vi "torque-write (SubVI).vi"(10 "Torque":i16, 11 "ID":u8) -> (3 "result string":string)   [LabVIEW 2017]
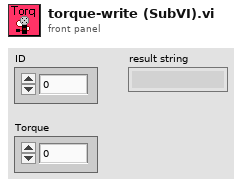
[diagram p1: front panel]
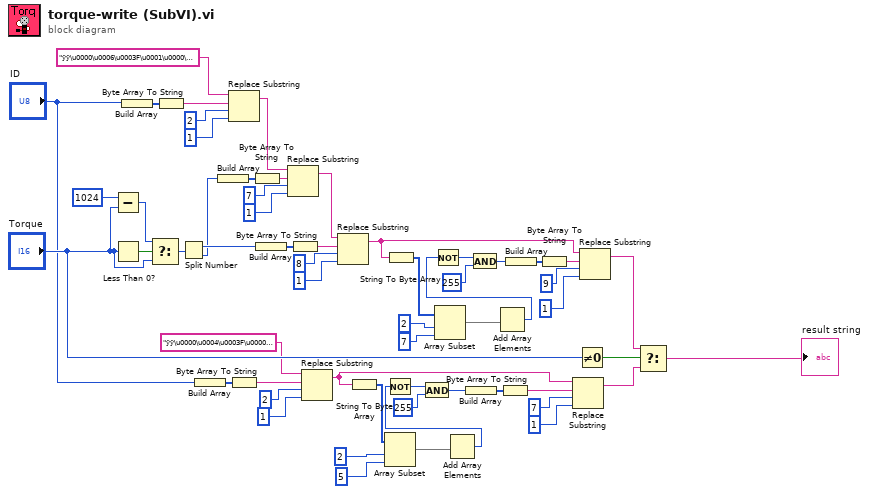
[diagram p0: block diagram]
diagram:
  n1 = Subtract(x=i16 1024, y="Torque") -> (x-y=w34:i16)
  n2 = Less Than 0?(x="Torque") -> (x < 0?=w29:bool)
  n3 = Build Array("ID") -> (w9:u8[])
  n4 = Select(t=w34, s=w29, f="Torque") -> (s? t:f=w31:i16)
  n5 = Byte Array To String(unsigned byte array=w9) -> (string=w8:string)
  n6 = Split Number(x=w31) -> (hi(x)=w33:u8, lo(x)=w32:u8)
  n7 = Build Array("ID") -> (w49:u8[])
  n8 = Build Array(w32) -> (w13:u8[])
  n9 = Replace Substring(2:1 ("length (len. of substring)"), 3:2 ("offset (0)"), 4:w8, 5:"ÿÿ\u0000\u0006\u0003F\u0001\u0000\u0000\u0000" ("string")) -> (1:w16:string)  [unwired: 1 out]
  n10 = Byte Array To String(unsigned byte array=w49) -> (string=w50:string)
  n11 = Byte Array To String(unsigned byte array=w13) -> (string=w12:string)
  n12 = Build Array(w33) -> (w4:u8[])
  n13 = Replace Substring(2:1 ("length (len. of substring)"), 3:7 ("offset (0)"), 4:w12, 5:w16) -> (1:w2:string)  [unwired: 1 out]
  n14 = Byte Array To String(unsigned byte array=w4) -> (string=w3:string)
  n15 = Replace Substring(2:1 ("length (len. of substring)"), 3:2 ("offset (0)"), 4:w50, 5:"ÿÿ\u0000\u0004\u0003F\u0000\u0000" ("string")) -> (1:w52:string)  [unwired: 1 out]
  n16 = Replace Substring(2:1 ("length (len. of substring)"), 3:8 ("offset (0)"), 4:w3, 5:w2) -> (1:w1:string)  [unwired: 1 out]
  n17 = String To Byte Array(string=w52) -> (unsigned byte array=w39:u8[])
  n18 = Array Subset(array=w39, index=2, length=5) -> (w36:u8[])
  n19 = String To Byte Array(string=w1) -> (unsigned byte array=w24:u8[])
  n20 = Array Subset(array=w24, index=2, length=7) -> (w27:u8[])
  n21 = Add Array Elements(numeric array=w36) -> (sum=w35:u8)
  n22 = Not(x=w35) -> (.not. x?=w46:u8)
  n23 = And(x=w46, y=u8 255) -> (x .and. y?=w40:u8)
  n24 = Build Array(w40) -> (w43:u8[])
  n25 = Add Array Elements(numeric array=w27) -> (sum=w28:u8)
  n26 = Not(x=w28) -> (.not. x?=w17:u8)
  n27 = And(x=w17, y=u8 255) -> (x .and. y?=w23:u8)
  n28 = Byte Array To String(unsigned byte array=w43) -> (string=w44:string)
  n29 = Build Array(w23) -> (w20:u8[])
  n30 = Byte Array To String(unsigned byte array=w20) -> (string=w19:string)
  n31 = Replace Substring(2:1 ("length (len. of substring)"), 3:7 ("offset (0)"), 4:w44, 5:w52) -> (1:w56:string)  [unwired: 1 out]
  n32 = Not Equal To 0?(x="Torque") -> (x != 0?=w55:bool)
  n33 = Replace Substring(2:1 ("length (len. of substring)"), 3:9 ("offset (0)"), 4:w19, 5:w1) -> (1:w57:string)  [unwired: 1 out]
  n34 = Select(t=w57, s=w55, f=w56) -> (s? t:f=→"result string":string)
